vi "Enviar_datosTest_Arduino.vi"(8 "error in (no error)":errorcluster, 10 "TEST ASICS INPUT":T1={"COORD. IN X"=0, "COORD IN Y"=0, "COORD OK X"=0, "COORD OK Y"=0, "COORD NOK X"=0, "COORD NOK Y"=0, "NºASICS A TESTEAR"=1, "SELECCIÓN DE TEST"=enum."TEST ASICS LST", "CUENTA ASICS"=0, "OPERADOR"="Javier Morales"}, 11 "VISA resource name":refnum<visa-resource-name>) -> (0 "error IO":errorcluster)   [LabVIEW 2019]
uses:
  Type_defs/INPUT TEST.ctl
  <vilib>/Utility/error.llb/Error Cluster From Error Code.vi
  <vilib>/ErrorRing/Error Ring.xnode
panel:
  out "trama datos":string
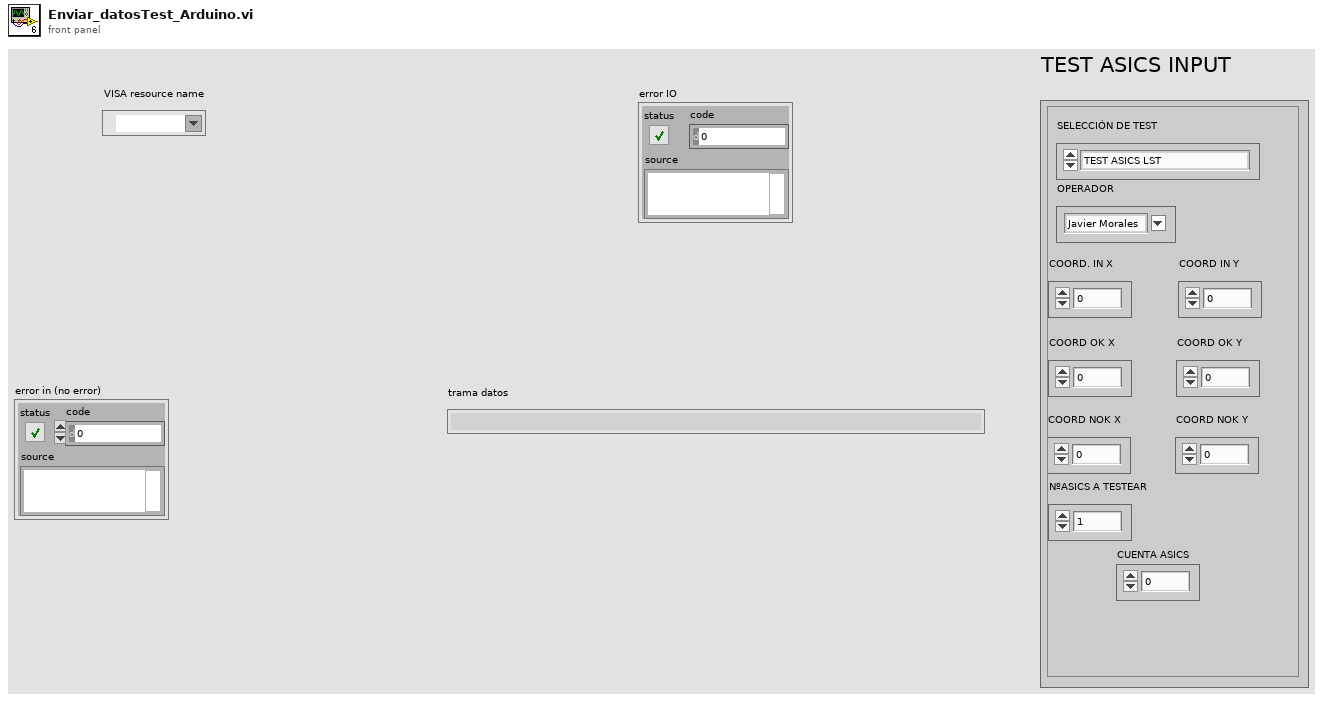
[diagram p1: front panel]
types:
  T1 = typedef "INPUT TEST.ctl" = cluster{"COORD. IN X":u16, "COORD IN Y":u16, "COORD OK X":u16, "COORD OK Y":u16, "COORD NOK X":u16, "COORD NOK Y":u16, "NºASICS A TESTEAR":u32, "SELECCIÓN DE TEST":enum16{"TEST ASICS LST"}, "CUENTA ASICS":u32, "OPERADOR":string}
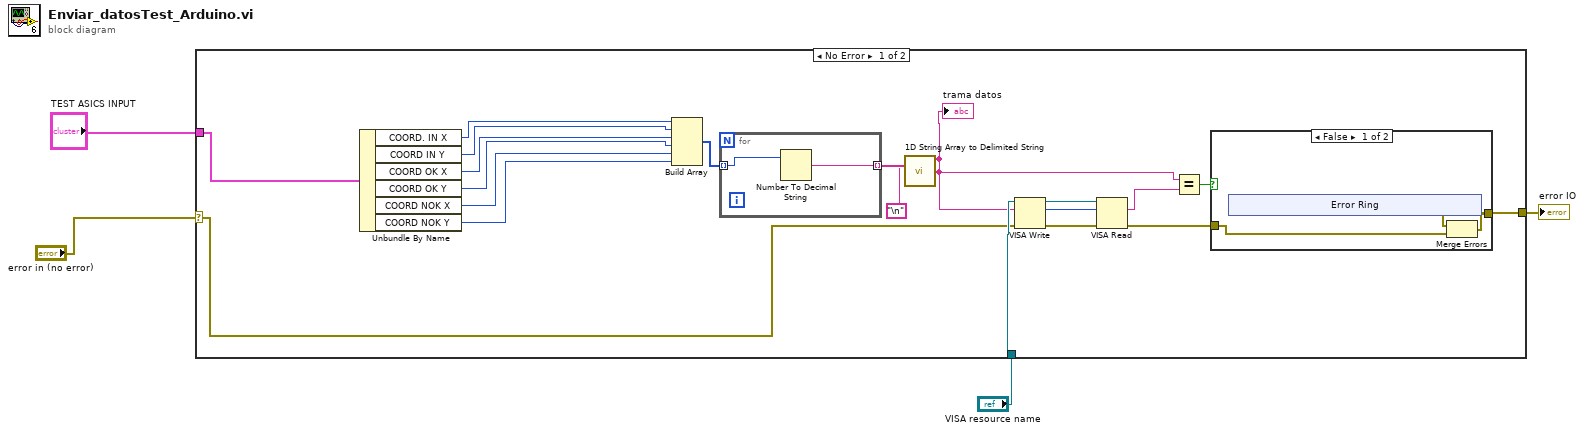
[diagram p0: block diagram]
diagram:
  n1 = case shown="No Error" "error in (no error)" {
    selector: "error in (no error)" -> [w20 w36]
    tunnel: "TEST ASICS INPUT" -> [w11 _]
    tunnel: "VISA resource name" -> [w21 _]
    tunnel: [w13 w36] -> w2
    frame No Error {
      n2 = Unbundle By Name(w11) -> ("COORD. IN X"=w10:u16, "COORD IN Y"=w9:u16, "COORD OK X"=w8:u16, "COORD OK Y"=w7:u16, "COORD NOK X"=w6:u16, "COORD NOK Y"=w5:u16)
      n3 = Build Array(w10, w9, w8, w7, w6, w5) -> (w24:u16[])
      n4 = for {
        tunnel: w24 -> [w34] mode=indexing
        tunnel: [w35] -> w23 mode=indexing
        n5 = Number To Decimal String(number=w34) -> (decimal integer string=w35:string)  [unwired: 1 in]
      }
      n6 = call <vilib>:"1D String Array to Delimited String.vi"("delimiter"="\n", "string array"=w23) -> ("delimited string"=w16:string)  [unwired: 9 in]
      "trama datos" <- w16
      n7 = VISA Write(VISA resource name=w21, write buffer=w16, error in (no error)=w20) -> (VISA resource name out=w18:refnum<visa-resource-name>, return count=w17:u32, error out=w19:errorcluster)
      n8 = VISA Read(VISA resource name=w18, byte count=w17, error in (no error)=w19) -> (read buffer=w15:string, error out=w12:errorcluster)  [unwired: 2 out]
      n9 = Equal?(x=w16, y=w15) -> (x = y?=w14:bool)
      n10 = case shown="False" w14 {
        tunnel: [w27 w33] -> w13
        tunnel: w12 -> [w25 w33]
        frame False {
          n11 = xnode "Error Ring"() -> ("error out"=w26:errorcluster)
          n12 = Merge Errors(w26, w25) -> (w27:errorcluster)
        }
        frame True {
        }
      }
    }
    frame Error {
    }
  }
  "error IO" <- w2
